vi "New Section.vi"(4 "Property Values":variant[](array[variant]), 6 "Property names":string[](array[string]), 8 "error in (no error)":errorcluster, 10 "TypeGUID":string, 11 "Name":string) -> (0 "error out":errorcluster, 3 "Section Reference in":u64 format="%.0x")   [LabVIEW 2013, in "Hierarchy Framework.lvlib" / "Section.lvclass"]
doc: "Create a new root <b>Section</b>."
uses:
  Section.lvclass
  Generic/Generic.lvclass
  Item/Item.lvclass
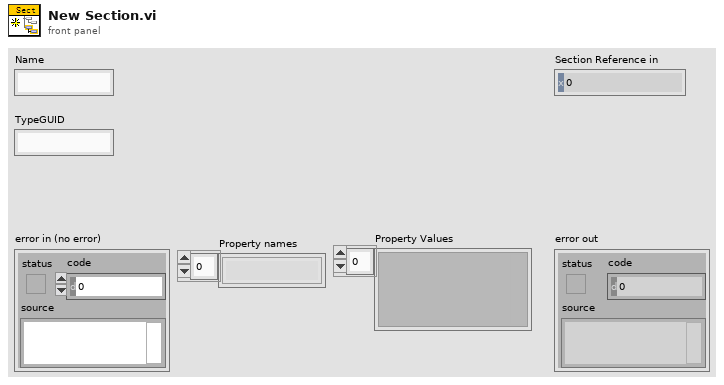
[diagram p1: front panel]
types:
  T1 = typedef "Hierarchy Framework.lvlib/Item.lvclass/Item Reference.ctl" = u64
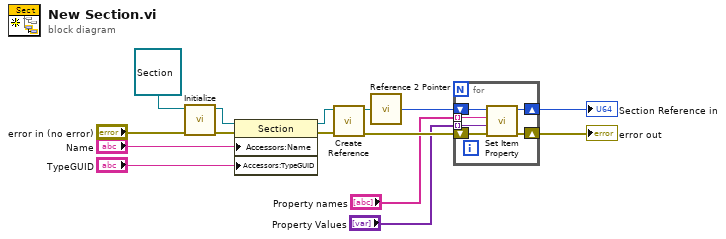
[diagram p0: block diagram]
diagram:
  n1 = call-dynamic "Initialize.vi"("error in (no error)"="error in (no error)", "Section输入"=refnum<class "Section.lvclass"> refnum ("Framework.lvlib:Section")) -> ("error out"=w13:errorcluster, "Section输出"=w15:refnum<class "Section.lvclass">)  [unwired: 8 in]
  n2 = property class="Section"(reference=w15, error in=w13, "Accessors:Name"="Name", "Accessors:TypeGUID"="TypeGUID") -> (reference out=w14:refnum<class "Section.lvclass">, error out=w10:errorcluster)
  n3 = call "Create Reference.vi"("error in (no error)"=w10, "Generic"=w14) -> ("error out"=w5:errorcluster, "Generic Reference"=w12:refnum<data-value>)  [unwired: 8 in]
  n4 = call "Reference 2 Pointer.vi"("Generic Reference"=w12) -> ("Pointer"=w6:u64)  [unwired: 1 out]
  n5 = for {
    shift-right: [w19] -> w4
    shift-left: w6 -> [w21]
    shift-right: [w18] -> w3
    shift-left: w5 -> [w20]
    tunnel: "Property names" -> [w17] mode=indexing
    tunnel: "Property Values" -> [w16] mode=indexing
    n6 = call "Set Item Property.vi"("error in (no error)"=w20, "Value"=w16, "Property Name"=w17, "Item Reference in"=w21) -> ("error out"=w18:errorcluster, "Item Reference out"=w19:T1)  [unwired: 5 in, 1 out]
  }
  "error out" <- w3
  "Section Reference in" <- w4
